vi "Dispose.vi"(8 "error in (no error)":errorcluster, 11 "Maze":refnum<class "Maze.lvclass">) -> (0 "error out":errorcluster)   [LabVIEW 2020, in "Maze.lvclass"]
uses:
  Maze.lvclass
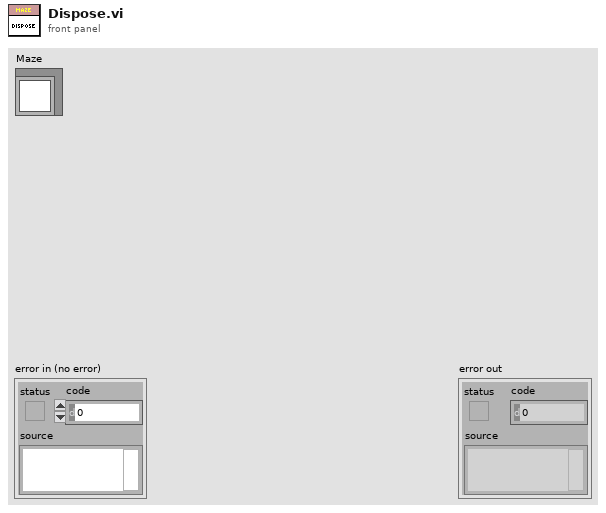
[diagram p1: front panel]
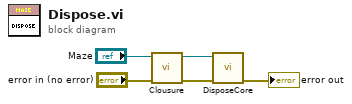
[diagram p0: block diagram]
diagram:
  n1 = call-dynamic "Clousure.vi"("error in (no error)"="error in (no error)", "Maze"="Maze") -> ("error out"=w2:errorcluster, "Maze"=w1:refnum<class "Maze.lvclass">)  [unwired: 8 in]
  n2 = call-dynamic "DisposeCore.vi"("error in (no error)"=w2, "Maze"=w1) -> ("error out"=→"error out":errorcluster)  [unwired: 8 in, 1 out]
